vi "ClaerNullStringArray.vi"(1 "Array in":string[](array[string])) -> (15 "Array out":string[](array[string]))   [LabVIEW 2015]
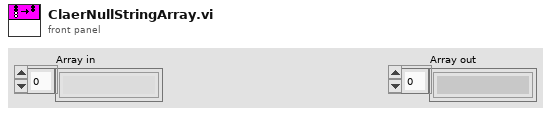
[diagram p1: front panel]
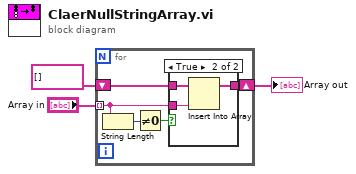
[diagram p0: block diagram]
diagram:
  n1 = for {
    tunnel: "Array in" -> [w6] mode=indexing
    shift-right: [w7] -> w1
    shift-left: string[] [] -> [w8]
    n2 = String Length(string=w6) -> (length=w4:i32)
    n3 = Not Equal To 0?(x=w4) -> (x != 0?=w5:bool)
    n4 = case shown="True" w5 {
      tunnel: w6 -> [_ w12]
      tunnel: w8 -> [w9 w11]
      tunnel: [w9 w10] -> w7
      frame False {
      }
      frame True {
        n5 = Insert Into Array(array=w11, new element=w12) -> (w10:string[])  [unwired: 1 in]
      }
    }
  }
  "Array out" <- w1
